vi "Initialize AI Task.vi"(8 "error in (no error)":errorcluster, 11 "BNT_ULx-MCSV-I in":refnum<class "BNT_ULx-MCSV-I.lvclass">) -> (0 "error out":errorcluster, 3 "AI ULx Task":refnum<k24>)   [LabVIEW 2020, in "BNT_ULx.lvlib" / "BNT_ULx-MCSV-I.lvclass"]
doc: "Initialize DAQmx Analog Input task. Every derived class needs to start the task on its own.\n\n<b>Default Implementation:</b> Analog Input Current\n\nThis dynamic dispatch VI can be overritten by derived classes to implement other analog input tasks."
uses:
  BNT_ULx-MCSV-I.lvclass
  C:/User/Brand/LVP/CSPP/CSPP-Template/Packages/CSPP_Core/Actors/CSPP_BaseActor/CSPP_BaseActor.lvclass
  C:/User/Brand/LVP/CSPP/CSPP-Template/Packages/BNT_ULx/BNT_ULx-MCSV/BNT_ULx-MCSV/BNT_ULx-MCSV.lvclass
  C:/Program Files (x86)/National Instruments/LabVIEW 2020/vi.lib/ULx/ULx_LV.dll
  Program Files (x86)/National Instruments/LabVIEW 2020/vi.lib/ULx/ULx_LV.dll
  CSPP_Core/Actors/CSPP_BaseActor/CSPP_BaseActor.lvclass/CSPP_BaseActor.ctl
  BNT_ULx-MCSV-I.lvclass/BNT_ULx-MCSV-I.ctl
  BNT_ULx-MCSV/BNT_ULx-MCSV.lvclass/BNT_ULx-MCSV.ctl
  CSPP_Core/Actors/CSPP_BaseActor/Read Object Name.vi
  Read External Shunt Resistor Value.vi
  BNT_ULx-MCSV/Read AI Terminal Configuration.vi
  BNT_ULx-MCSV/Read AI Min.vi
  BNT_ULx-MCSV/Read AI Max.vi
  BNT_ULx-MCSV/Read AI ULx Physical Channels.vi
  Read Shunt Resistor Location.vi
  <vilib>/ULx/Create Channel.llb/ULx Create Channel (AI-Current-Basic).vi
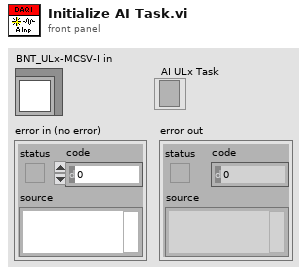
[diagram p1: front panel]
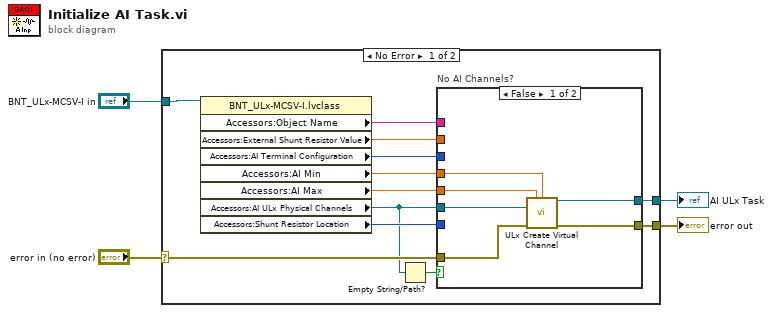
[diagram p0: block diagram]
diagram:
  n1 = case shown="No Error" "error in (no error)" {
    selector: "error in (no error)" -> [w16 w24]
    tunnel: [w8 w24] -> w1
    tunnel: "BNT_ULx-MCSV-I in" -> [w15 _]
    tunnel: [w9 _] -> w2
    frame No Error {
      n2 = property class="BNT_ULx-MCSV-I.lvclass"(reference=w15) -> ("Accessors:Object Name"=w7:string, "Accessors:External Shunt Resistor Value"=w11:dbl[unit], "Accessors:AI Terminal Configuration"=w12:i32, "Accessors:AI Min"=w13:dbl, "Accessors:AI Max"=w14:dbl, "Accessors:AI ULx Physical Channels"=w6:refnum<k21>, "Accessors:Shunt Resistor Location"=w10:i32)  [unwired: 1 in, 2 out]
      n3 = Empty String/Path?(string/path=w6) -> (empty?=w5:bool)
      n4 = case "No AI Channels?" shown="False" w5 {
        tunnel: w16 -> [w22 w23]
        tunnel: w6 -> [w19 _]
        tunnel: w14 -> [w17 _]
        tunnel: w13 -> [w18 _]
        tunnel: w12 -> [_ _]
        tunnel: w11 -> [_ _]
        tunnel: w10 -> [_ _]
        tunnel: [w20 _] -> w9
        tunnel: [w21 w23] -> w8
        tunnel: w7 -> [_ _]
        frame False {
          n5 = call-poly <vilib>:"ULx Create Virtual Channel.vi"("maximum value"=w17, "minimum value"=w18, "physical channels"=w19, "error in"=w22) -> ("task out"=w20:refnum<k24>, "error out"=w21:errorcluster)  [unwired: 10 in]
        }
        frame True {
        }
      }
    }
    frame Error {
    }
  }
  "error out" <- w1
  "AI ULx Task" <- w2
